vi "Find Coordinate.vi"(5 "Bounding Box":cluster{dbl, dbl, dbl, dbl, dbl}, 6 "Detector Interval":i32=3, 7 "Subset Length":i32=3, 8 "String":string="X", 9 "method":u16(ring)=1 items=["2nd Order Central", "4th Order Central", "Forward", "Backward"], 10 "Search Lines Information 2":T1[](array[typedef]) {"Edge Info"."Distance (Real-World)" format="%.2f"; "Edge Info"."Location (Real-World)"."Y" format="%.2g"; "Edge Info"."Location (Real-World)"."X" format="%.2f"; "Edge Info"."Noise" format="%.2f"; "Edge Info"."Location (Pixel)"."Y" format="%.2g"; "Edge Info"."Location (Pixel)"."X" format="%.2f"; "Edge Info"."Strength" format="%.2f"; "Edge Info"."Distance (Pixel)" format="%.2f"}, 11 "Search Lines Information":T1[](array[typedef]) {"Edge Info"."Distance (Real-World)" format="%.2f"; "Edge Info"."Location (Real-World)"."Y" format="%.2g"; "Edge Info"."Location (Real-World)"."X" format="%.2f"; "Edge Info"."Noise" format="%.2f"; "Edge Info"."Location (Pixel)"."Y" format="%.2g"; "Edge Info"."Location (Pixel)"."X" format="%.2f"; "Edge Info"."Strength" format="%.2f"; "Edge Info"."Distance (Pixel)" format="%.2f"}) -> (3 "Centerpoint 3":cluster{dbl, dbl})   [LabVIEW 2018]
uses:
  <vilib>/vision/Measure.llb/Search Line.ctl
  <vilib>/vision/Measure.llb/Edge New.ctl
  <vilib>/Analysis/baseanly.llb/Mean (DBL).vi
  <vilib>/Analysis/1siggen.llb/Ramp Pattern by Delta.vi
  <vilib>/Analysis/NI_AALPro.lvlib
  <vilib>/Analysis/NI_AALBase.lvlib
panel:
  out "output cluster":cluster{"Ramp Pattern":dbl[], "dX/dt":dbl[]}(graph)
  out "dX/dt":dbl[](array[numeric])
  out "Averaged Values":dbl[][](array[numeric])
  out "Array 2":dbl[](array[numeric])
  out "Array":dbl[](array[numeric])
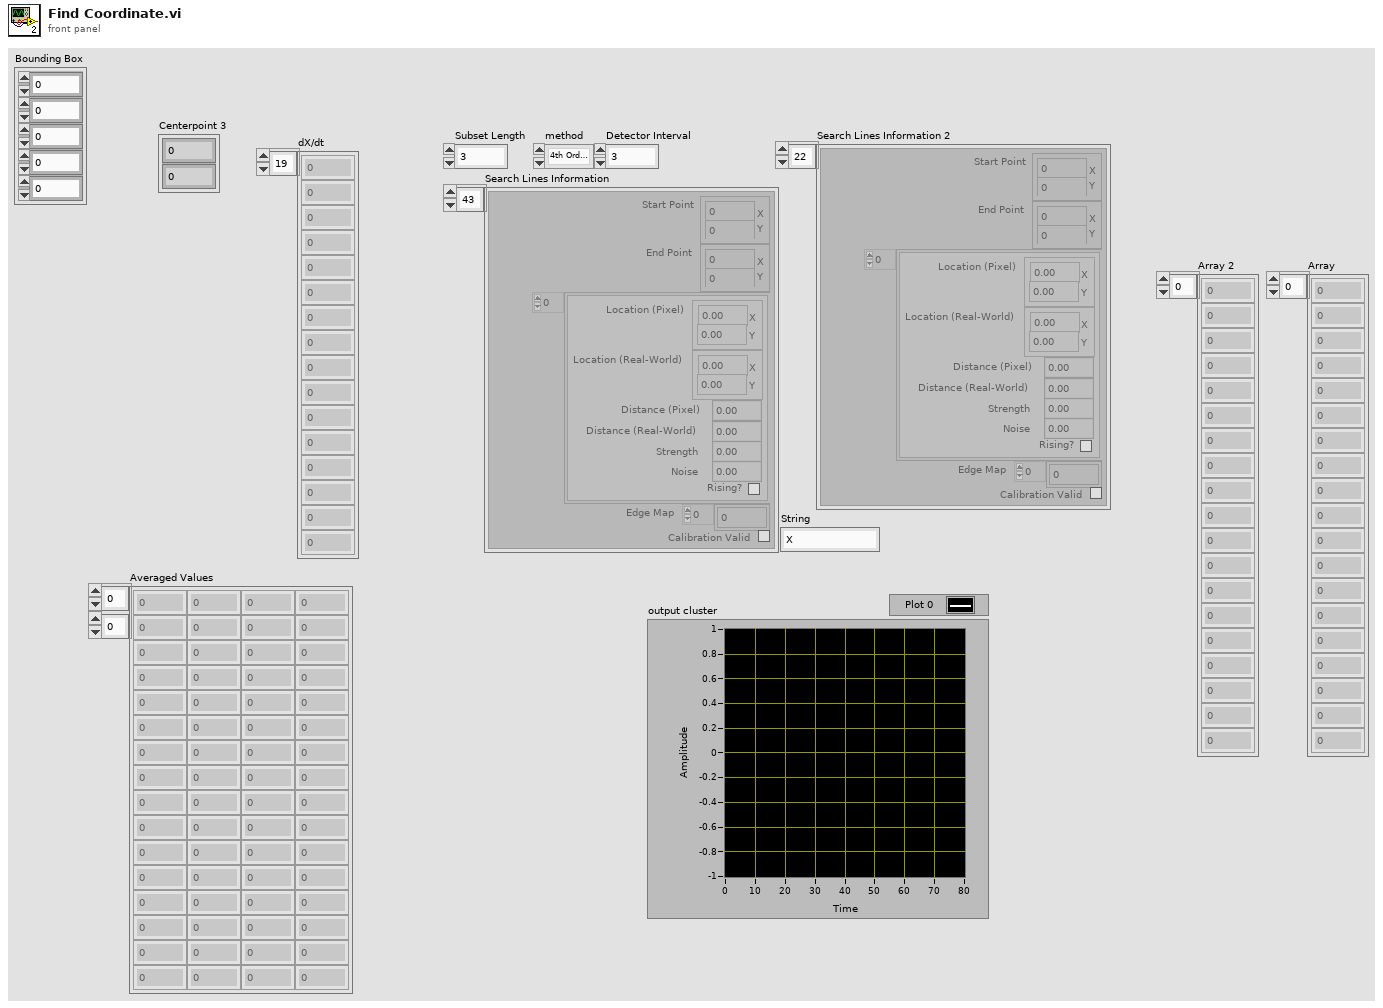
[diagram p1: front panel]
types:
  T1 = typedef "Search Line.ctl" = cluster{"Start Point":cluster{"X":sgl, "Y":sgl}, "End Point":cluster{"X":sgl, "Y":sgl}, "Edge Info":T2[], "Edge Map":dbl[], "Calibration Valid":bool}
  T2 = typedef "Edge New.ctl" = cluster{"Location (Pixel)":cluster{"X":sgl, "Y":sgl}, "Location (Real-World)":cluster{"X":sgl, "Y":sgl}, "Distance (Pixel)":dbl, "Distance (Real-World)":dbl, "Strength":dbl, "Noise":dbl, "Rising?":bool}
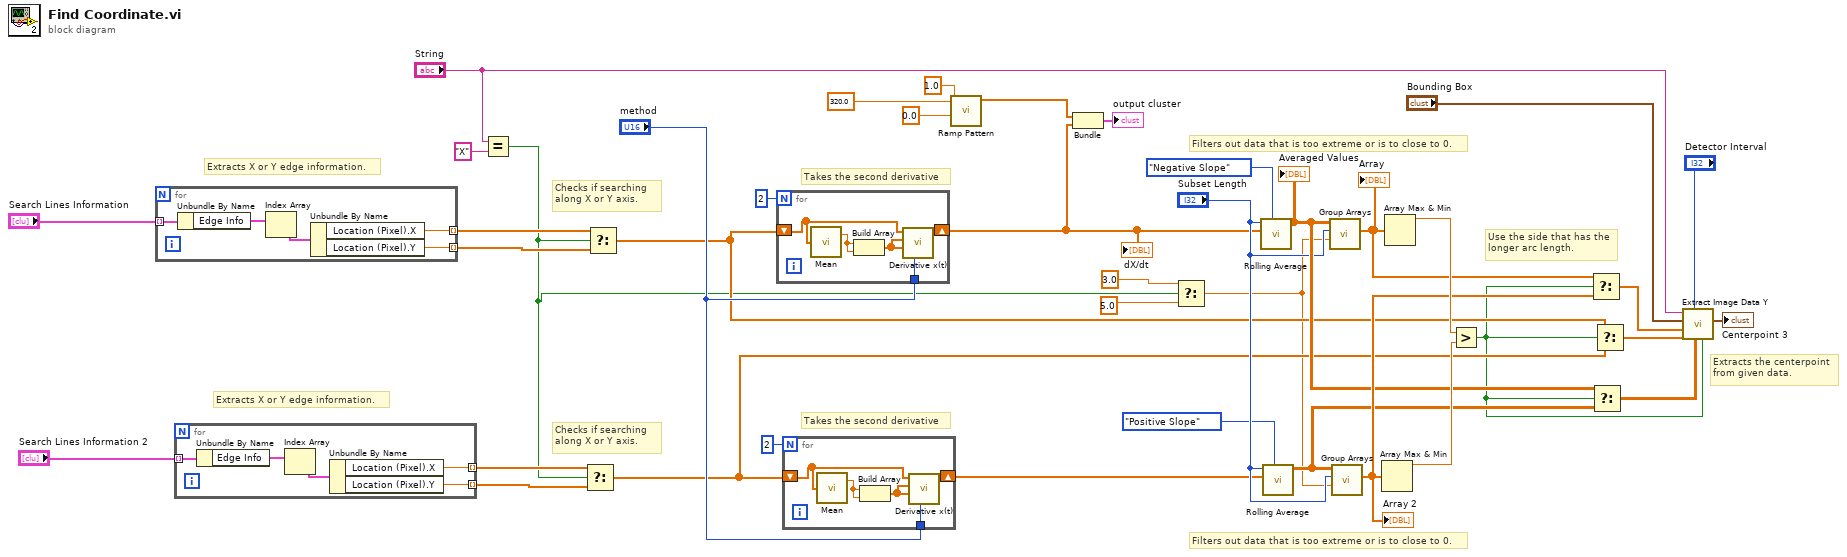
[diagram p0: block diagram]
diagram:
  # "Extracts the centerpoint\nfrom given data."
  # "Use the side that has the\nlonger arc length."
  # "Filters out data that is too extreme or is to close to 0."
  # "Filters out data that is too extreme or is to close to 0."
  # "Takes the second derivative"
  # "Takes the second derivative"
  # "Checks if searching \nalong X or Y axis."
  # "Checks if searching \nalong X or Y axis."
  # "Extracts X or Y edge information."
  # "Extracts X or Y edge information."
  n1 = for {
    tunnel: "Search Lines Information" -> [w45] mode=indexing
    tunnel: [w42] -> w21 mode=indexing
    tunnel: [w41] -> w20 mode=indexing
    n2 = Unbundle By Name(w45) -> ("Edge Info"=w44:T2[])
    n3 = Index Array(array=w44) -> (element=w43:T2)  [unwired: 1 in]
    n4 = Unbundle By Name(w43) -> ("Location (Pixel).X"=w42:sgl, "Location (Pixel).Y"=w41:sgl)
  }
  n5 = for {
    tunnel: "Search Lines Information 2" -> [w50] mode=indexing
    tunnel: [w47] -> w19 mode=indexing
    tunnel: [w46] -> w18 mode=indexing
    n6 = Unbundle By Name(w50) -> ("Edge Info"=w49:T2[])
    n7 = Index Array(array=w49) -> (element=w48:T2)  [unwired: 1 in]
    n8 = Unbundle By Name(w48) -> ("Location (Pixel).X"=w47:sgl, "Location (Pixel).Y"=w46:sgl)
  }
  n9 = Equal?(x="String", y="X") -> (x = y?=w5:bool)
  n10 = Select(t=w19, s=w5, f=w18) -> (s? t:f=w12:sgl[])
  n11 = Select(t=w21, s=w5, f=w20) -> (s? t:f=w10:sgl[])
  n12 = for {
    N: 2 -> [_]
    shift-right: [w55] -> w9
    shift-left: w10 -> [w54]
    tunnel: "method" -> [w51]
    n13 = call-poly <vilib>:"Mean.vi"("X"=w54) -> ("mean"=w53:dbl)  [unwired: 1 out]
    n14 = Build Array(w53, w53) -> (w52:dbl[])
    n15 = call <vilib>:"Derivative x(t).vi"("method"=w51, "Final Condition"=w52, "Initial Condition"=w52, "X"=w54) -> ("dX/dt"=w55:dbl[])  [unwired: 6 in, 1 out]
  }
  "dX/dt" <- w9
  n16 = for {
    N: 2 -> [_]
    tunnel: "method" -> [w59]
    shift-right: [w60] -> w11
    shift-left: w12 -> [w58]
    n17 = call-poly <vilib>:"Mean.vi"("X"=w58) -> ("mean"=w57:dbl)  [unwired: 1 out]
    n18 = Build Array(w57, w57) -> (w56:dbl[])
    n19 = call <vilib>:"Derivative x(t).vi"("method"=w59, "Final Condition"=w56, "Initial Condition"=w56, "X"=w58) -> ("dX/dt"=w60:dbl[])  [unwired: 6 in, 1 out]
  }
  n20 = call-poly <vilib>:"Ramp Pattern.vi"("start"=0.0, "end"=320.0, "delta"=1.0) -> ("Ramp Pattern"=w16:dbl[])  [unwired: 6 in, 2 out]
  n21 = Bundle("Ramp Pattern"=w16, "dX/dt"=w9) -> (→"output cluster":cluster{"Ramp Pattern":dbl[], "dX/dt":dbl[]})  [unwired: 1 in]
  n22 = Select(t=3.0, s=w5, f=5.0 ("Grouping Size")) -> (s? t:f=w4:dbl)
  n23 = call "Rolling Average.vi"("Enum"=enum16{"Positive Slope", "Negative Slope"}."Negative Slope", "Filtered X"=w9, "Subset Length"="Subset Length") -> ("Averaged Values"=w34:dbl[][])  [unwired: 8 in]
  "Averaged Values" <- w34
  n24 = call "Rolling Average.vi"("Enum"=enum16{"Positive Slope", "Negative Slope"}."Positive Slope", "Filtered X"=w11, "Subset Length"="Subset Length") -> ("Averaged Values"=w33:dbl[][])  [unwired: 8 in]
  n25 = call "Group Arrays.vi"("Grouping Size"=w4, "length"="Subset Length", "Averaged Values"=w34) -> ("Array"=w36:dbl[])  [unwired: 8 in]
  "Array" <- w36
  n26 = call "Group Arrays.vi"("Grouping Size"=w4, "length"="Subset Length", "Averaged Values"=w33) -> ("Array"=w35:dbl[])  [unwired: 8 in]
  "Array 2" <- w35
  n27 = Array Max & Min(array=w35) -> (max value=w37:dbl)  [unwired: 3 out]
  n28 = Array Max & Min(array=w36) -> (max value=w38:dbl)  [unwired: 3 out]
  n29 = Greater?(x=w38, y=w37) -> (0:w1:bool)
  n30 = Select(t=w36, s=w1, f=w35) -> (s? t:f=w32:dbl[])
  n31 = Select(t=w34, s=w1, f=w33) -> (s? t:f=w30:dbl[][])
  n32 = Select(t=w10, s=w1, f=w12) -> (s? t:f=w31:sgl[])
  n33 = call "Extract Image Data Y.vi"("Negative Slope"=w1, "Averaged Values"=w30, "Detector Interval"="Detector Interval", "Original values"=w31, "Grouped Arrays"=w32, "Bounding Box"="Bounding Box", "String"="String") -> ("Centerpoint"=→"Centerpoint 3":cluster{dbl, dbl})  [unwired: 4 in]
